vi "MMinStatus.vi"(0 "VisaCluster":T1, 11 "error in (no error)":errorcluster) -> (4 "VisaCluster":T1, 8 "Answer":string, 15 "error out":errorcluster)   [LabVIEW 2014, in "FH 55.lvlib"]
doc: "Dieses Vi gibt den minimalen Messwert aus dem Gerät zurück.\n\nThis vi returns the minimum measurement from the instrument."
uses:
  FH 55.lvlib
  TypeDef/VisaCluster.ctl
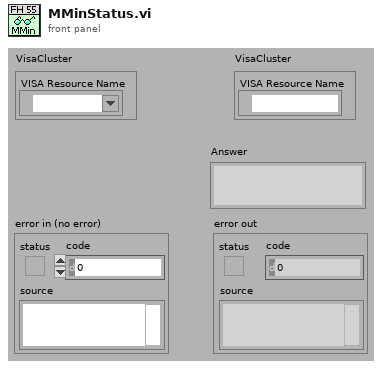
[diagram p1: front panel]
types:
  T1 = typedef "FH 55.lvlib/VisaCluster.ctl" = cluster{"VISA Resource Name":refnum<visa-resource-name>}
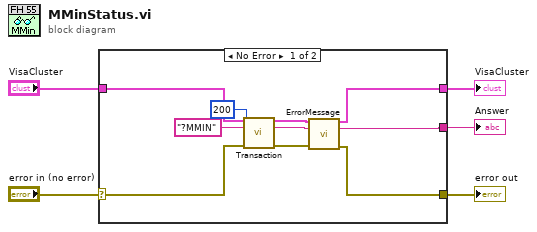
[diagram p0: block diagram]
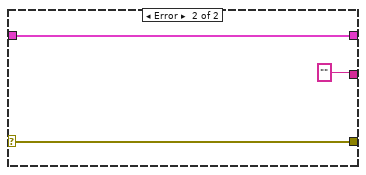
[diagram p2: hidden frame]
diagram:
  n1 = case shown="No Error" "error in (no error)" {
    selector: "error in (no error)" -> [w13 w17]
    tunnel: "VisaCluster" -> [w14 w18]
    tunnel: [w9 w18] -> w1
    tunnel: [w11 w17] -> w3
    tunnel: [w7 ""] -> w2
    frame No Error {
      n2 = call "Transaction.vi"("VisaCluster"=w14, "Command"="?MMIN", "Time (150) ms"=u32 200, "error in (no error)"=w13) -> ("VisaCluster"=w10:T1, "Answer"=w8:string, "error out"=w12:errorcluster)  [unwired: 8 in, 1 out]
      n3 = call "ErrorMessage.vi"("VisaCluster"=w10, "Message In"=w8, "error in (no error)"=w12) -> ("VisaCluster"=w9:T1, "Message Out"=w7:string, "error out"=w11:errorcluster)  [unwired: 10 in]
    }
    frame Error {
    }
  }
  "error out" <- w3
  "Answer" <- w2
  "VisaCluster" <- w1
